vi "Generate proto file.vi"(8 "error in":errorcluster, 9 "gRPC proto File Name":string, 10 "gRPC Service Name":string, 11 "PluginGenerator_MetaDataObj":refnum<class "PluginGenerator_MetaDataObj.lvclass">) -> (0 "error out":errorcluster, 2 "proto File Path":path, 3 "PluginGenerator_MetaDataObj out":refnum<class "PluginGenerator_MetaDataObj.lvclass">)   [LabVIEW 2021, in "Plugin Generator.lvlib"]
uses:
  Plugin Generator.lvlib
  PluginGenerator_MetaDataObj/PluginGenerator_MetaDataObj.lvclass
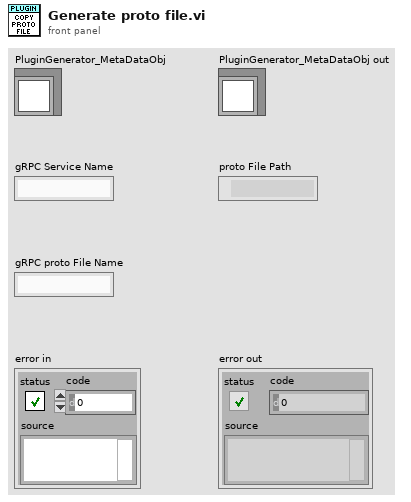
[diagram p1: front panel]
types:
  T1 = enum16{"open", "replace", "create", "open or create", "replace or create", "replace or create with confirmation"}
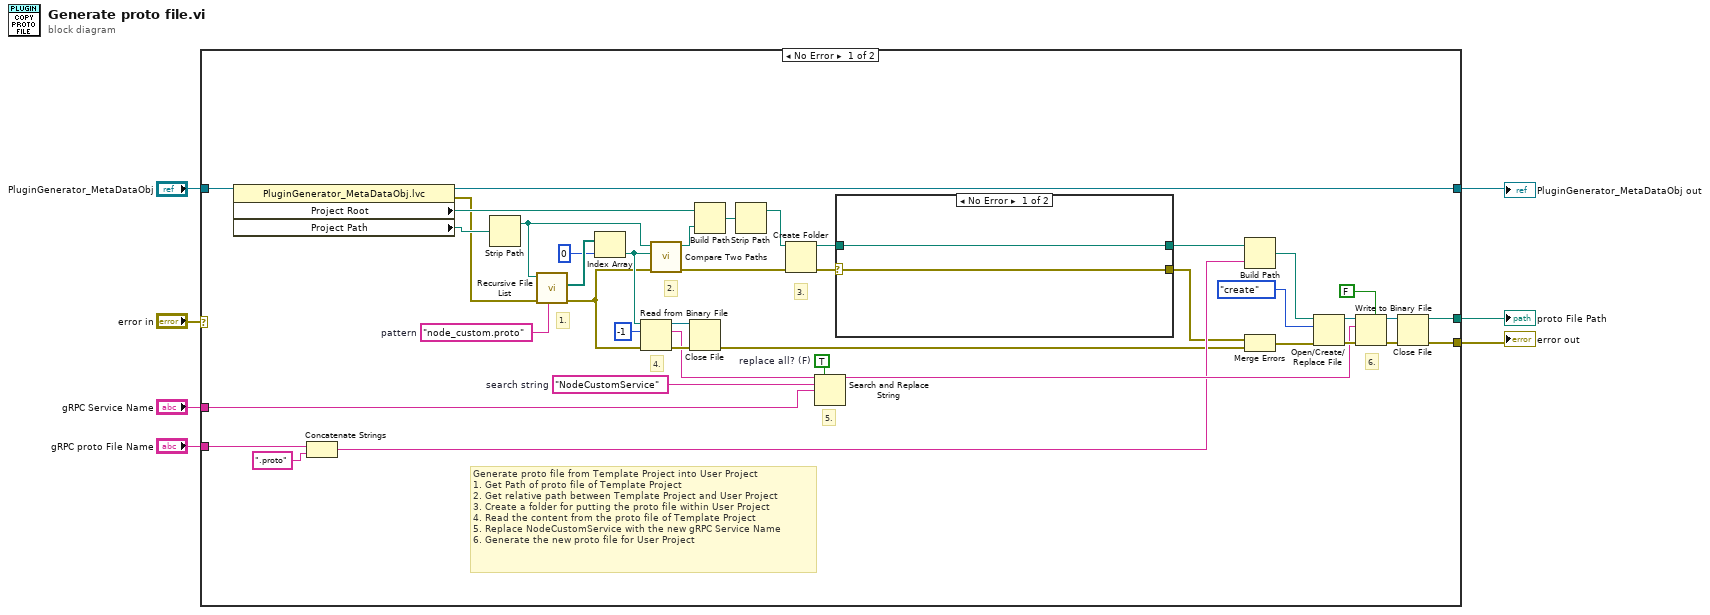
[diagram p0: block diagram]
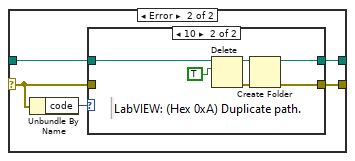
[diagram p2: hidden frame]
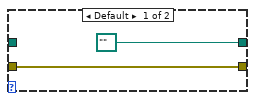
[diagram p3: hidden frame]
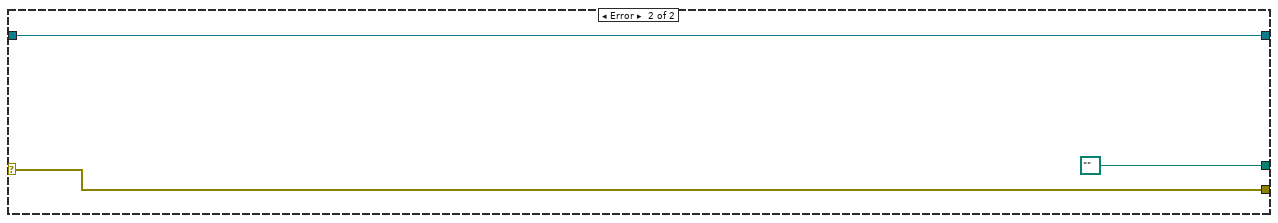
[diagram p4: hidden frame]
diagram:
  n1 = case shown="No Error" "error in" {
    selector: "error in" -> [_ w66]
    tunnel: "gRPC Service Name" -> [w29 _]
    tunnel: [w25 w66] -> w6
    tunnel: [w19 path "" ("path")] -> w5
    tunnel: "gRPC proto File Name" -> [w18 _]
    tunnel: "PluginGenerator_MetaDataObj" -> [w14 w65]
    tunnel: [w8 w65] -> w1
    frame No Error {
      w11 = TRUE  # replace all? (F)
      w36 = "NodeCustomService"  # search string
      w48 = "node_custom.proto"  # pattern
      # "6."
      # "5."
      # "4."
      # "3."
      # "2."
      # "1."
      # "Generate proto file from Template Project into User Project\n1. Get Path of proto file of Template Project\n2. Get relative path between Template Project and User Project\n3. Create a folder for putting the proto file within User Project\n4. Read the content from the proto file of Template Project\n5. Replace NodeCustomService with the new gRPC Service Name\n6. Generate the new proto file for User Project"
      n2 = property class="PluginGenerator_MetaDataObj.lvc"(reference=w14) -> (reference out=w8:refnum<class "PluginGenerator_MetaDataObj.lvclass">, error out=w9:errorcluster, "Project Root"=w13:path, "Project Path"=w12:path)  [unwired: 1 in]
      n3 = Concatenate Strings(w18, ".proto" ("string")) -> (w27:string)
      n4 = Strip Path(path=w12) -> (stripped path=w45:path)  [unwired: 1 out]
      n5 = call <vilib>:"Recursive File List.vi"("pattern"=w48, "error in (no error)"=w9, "Folder Path"=w45) -> ("error out"=w24:errorcluster, "All Files in Dir"=w47:path[])  [unwired: 4 in, 3 out]
      n6 = Index Array(array=w47, index=0) -> (element=w41:path)
      n7 = Read from Binary File(8:w24, 10:-1 ("count (1)"), 11:w41) -> (0:w39:errorcluster, 2:w37:string, 3:w38:refnum<file>)  [unwired: 3 in, 1 out]
      n8 = call <vilib>:"Compare Two Paths.vi"("error in (no error)"=w24, "Path 2"=w41, "Path 1"=w45) -> ("error out"=w42:errorcluster, "Relative Path from 1 to 2"=w44:path)  [unwired: 5 in, 2 out]
      n9 = Close File(refnum=w38, error in=w39) -> (error out=w23:errorcluster)  [unwired: 1 out]
      n10 = Build Path(base path=w13, name or relative path=w44) -> (appended path=w43:path)
      n11 = Strip Path(path=w43) -> (stripped path=w20:path)  [unwired: 1 out]
      n12 = Create Folder(path (use dialog)=w20, error in=w42) -> (created path=w16:path, error out=w17:errorcluster)  [unwired: 1 in, 1 out]
      n13 = Search and Replace String(replace all?=w11, input string=w37, search string=w36, replace string=w29) -> (result string=w31:string)  [unwired: 4 in, 3 out]
      n14 = case shown="No Error" w17 {
        selector: w17 -> [w50 w52]
        tunnel: [w50 w53] -> w15
        tunnel: w16 -> [w49 w54]
        tunnel: [w49 w51] -> w10
        frame No Error {
        }
        frame Error {
          n15 = Unbundle By Name(w52) -> ("code"=w55:i32)
          n16 = case shown="10" w55 {
            tunnel: w54 -> [_ w63]
            tunnel: [w57 w58] -> w53
            tunnel: w52 -> [w57 _]
            tunnel: [path "" ("created path") w59] -> w51
            frame Default {
            }
            frame 10 {
              n17 = Delete(path (use dialog)=w63, entire hierarchy (F)=TRUE) -> (deleted path=w60:path, error out=w61:errorcluster)  [unwired: 3 in, 1 out]
              n18 = Create Folder(path (use dialog)=w60, error in=w61) -> (created path=w59:path, error out=w58:errorcluster)  [unwired: 1 in, 1 out]
            }
          }
        }
      }
      n19 = Build Path(base path=w10, name or relative path=w27) -> (appended path=w26:path)
      n20 = Merge Errors(w15, w23) -> (w22:errorcluster)
      n21 = Open/Create/Replace File(file path (use dialog)=w26, error in=w22, operation (0:open)=T1."create") -> (refnum out=w35:refnum<file>, error out=w34:errorcluster)  [unwired: 3 in, 1 out]
      n22 = Write to Binary File(file (use dialog)=w35, data=w31, error in=w34, 5:FALSE ("prepend array or string size? (T)")) -> (refnum out=w33:refnum<file>, error out=w32:errorcluster)  [unwired: 2 in, 1 out]
      n23 = Close File(refnum=w33, error in=w32) -> (path=w19:path, error out=w25:errorcluster)
    }
    frame Error {
    }
  }
  "error out" <- w6
  "proto File Path" <- w5
  "PluginGenerator_MetaDataObj out" <- w1
